vi "Write IRuleFileParser.vi"(9 "IRuleFileParser":refnum<class "IRuleFileParser.lvclass">, 11 "CDependencyInspection in":refnum<class "CDependencyInspection.lvclass">) -> (3 "CDependencyInspection out":refnum<class "CDependencyInspection.lvclass">)   [LabVIEW 2020, in "DependencyInspection.lvlib" / "CDependencyInspection.lvclass"]
uses:
  CDependencyInspection.lvclass
  ExtensionInterfaces/IRuleFileParser/IRuleFileParser.lvclass
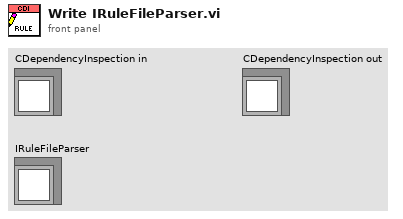
[diagram p1: front panel]
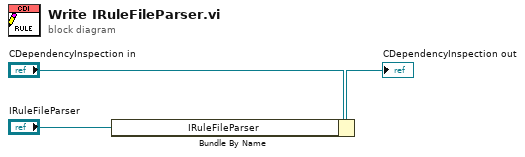
[diagram p0: block diagram]
diagram:
  n1 = Bundle By Name(cluster="CDependencyInspection in", "IRuleFileParser"="IRuleFileParser") -> (→"CDependencyInspection out":refnum<class "CDependencyInspection.lvclass">)
